vi "target.vi"() -> ()   [LabVIEW 2017]
panel:
  in  "stop":bool
  out "objreg":string
  in  "y":dbl
  in  "x":dbl
  in  "etl0":dbl
  in  "target":bool
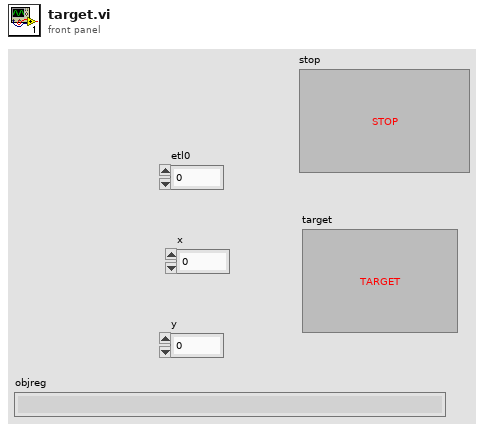
[diagram p1: front panel]
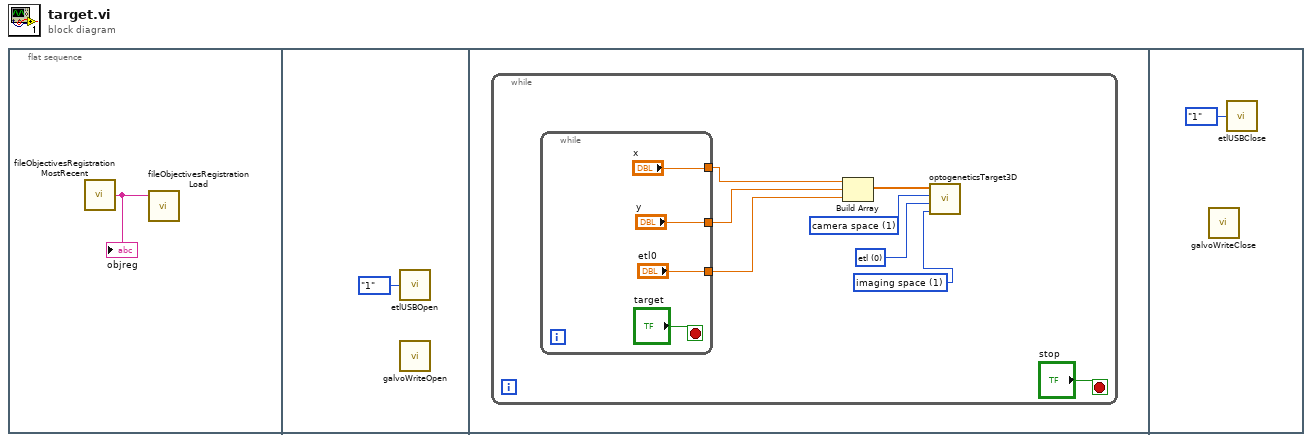
[diagram p0: block diagram]
diagram:
  n1 = flat-sequence {
    frame #0 {
      n2 = call "fileObjectivesRegistrationMostRecent.vi"() -> ("f"=w1:string)  [unwired: 1 in]
      "objreg" <- w1
      n3 = call "fileObjectivesRegistrationLoad.vi"("objectiveRegistrationFilePath"=w1) -> ()  [unwired: 3 in, 6 out]
    }
    frame #1 {
      n4 = call "etlUSBOpen.vi"("lens"=enum16{"0", "1"}."1") -> ()  [unwired: 1 in, 1 out]
      n5 = call "galvoWriteOpen.vi"() -> ()  [unwired: 12 in]
    }
    frame #2 {
      n6 = while {
        stop <- "stop" stop-if-true
        w7 = u16 1 items=["optogenetics space", "imaging space"] ("z mode")
        w8 = u16 0 items=["etl", "piezo"] ("z device")
        w9 = u16 1 items=["galvo space", "camera space"] ("xy mode")
        n7 = while {
          tunnel: ["x"] -> w6
          tunnel: ["y"] -> w5
          tunnel: ["etl0"] -> w4
          stop <- "target" stop-if-true
        }
        n8 = Build Array(w6, w5, w4) -> (w10:dbl[])
        n9 = call "optogeneticsTarget3D.vi"("z mode"=w7, "z device"=w8, "xy mode"=w9, "xyz"=w10) -> ()  [unwired: 1 in]
      }
    }
    frame #3 {
      n10 = call "galvoWriteClose.vi"() -> ()  [unwired: 12 in]
      n11 = call "etlUSBClose.vi"("lens"=enum16{"0", "1"}."1") -> ()  [unwired: 1 in]
    }
  }
